vi "PJVS.vi"(3 "Trim current (A) (+- 0.002)":dbl, 4 "Samples (2) (2 - 256)":i32=2 min=2 max=256, 5 "Frequency  (0 Hz) (0, 0.5 - 10e3)":dbl, 6 "Waveform (Sinewave)":T2, 7 "Voltage (0 V DC/RMS) (DC: +- 10.1, AC: 0 - 7.2)":dbl, 8 "error in (no error)":errorcluster) -> (0 "error out":errorcluster, 2 "PJVS Voltages":T1={"DC Voltage (S)"=nan, "AC Josephson Voltage RMS (V)"=nan, "Number of steps"=-1, "AC Voltages (V)"=[]} {"AC Voltages (V)" format="%#_10g"; "AC Josephson Voltage RMS (V)" format="%#_10g"; "DC Voltage (S)" format="%#_10g"})   [LabVIEW 2019, in "ACSVcontrol-driver.lvlib"]
doc: "Sets PJVS voltage(s). If frequency is nonzero, the AC mode is supposed. Samples sets the number of steps into which the waveform is divided. Output is a structure with DC voltage or AC voltages and steps."
uses:
  ACSVcontrol-driver.lvlib
  Type Definitions/Waveform.ctl
  Type Definitions/PJVS Voltages.ctl
  Private/Type definitions/Command.ctl
  Private/Type definitions/Status.ctl
  Private/Type definitions/Instruction.ctl
  Private/Globals.vi
  <vilib>/Utility/error.llb/Error Cluster From Error Code.vi
  <vilib>/ErrorRing/Error Ring.xnode
panel:
  in  "number format string":string="%.6f"
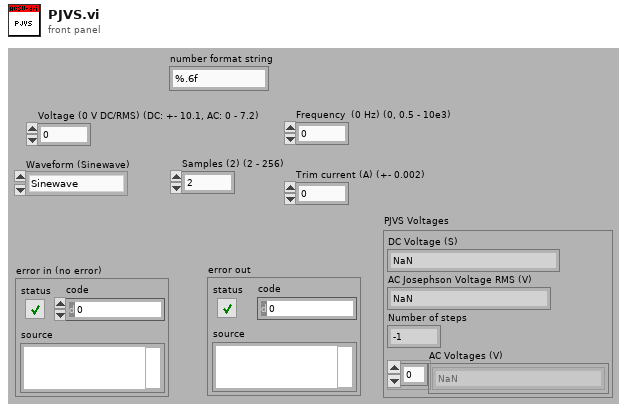
[diagram p1: front panel]
types:
  T1 = typedef "ACSVcontrol-driver.lvlib/PJVS Voltages.ctl" = cluster{"DC Voltage (S)":dbl, "AC Josephson Voltage RMS (V)":dbl, "Number of steps":i32, "AC Voltages (V)":dbl[]}
  T2 = typedef "ACSVcontrol-driver.lvlib/Waveform.ctl" = enum16{"Sinewave", "Triangle", "Sawtooth", "Rectangle", "Arbitrary"}
  T3 = typedef "ACSVcontrol-driver.lvlib/Status.ctl" = enum16{"waiting", "processing", "error command", "Set_PJVS-Done", "Set_Mux-Done", "Set_Mux-Error", "Set_57XX-Done", "Set_57XX-Error", "Set_Gen-Done", "Set_Gen-Error", "Set_Synthesizer-Done", "Set_Synthesizer-Error", "Read_Nano-Done", "Read_Sampler-Done", "Read_Sampler-Error", "Read_Sensors-Done"}
  T4 = typedef "ACSVcontrol-driver.lvlib/Command.ctl" = enum16{"Set_PJVS", "Set_Mux", "Set_57XX", "Set_Gen", "Set_Synthesizer", "Read_Nulldetector", "Read_Sampler", "Read_Sensors"}
  T5 = typedef "ACSVcontrol-driver.lvlib/Instruction.ctl" = enum16{"dummy - do not use", "Send Command", "Read Result", "Ask Status"}
  T6 = typedef "ACSVcontrol-driver.lvlib/Timeouts.ctl" = cluster{"TCP Read & Write (ms)":i32, "Sensors readout":i32, "PJVS setup":i32, "Nullmeter readout":i32, "Multiplexer setup":i32, "57XX setup":i32, "Generator setup":i32, "Synthesizer setup":i32, "Sampler readout":i32}
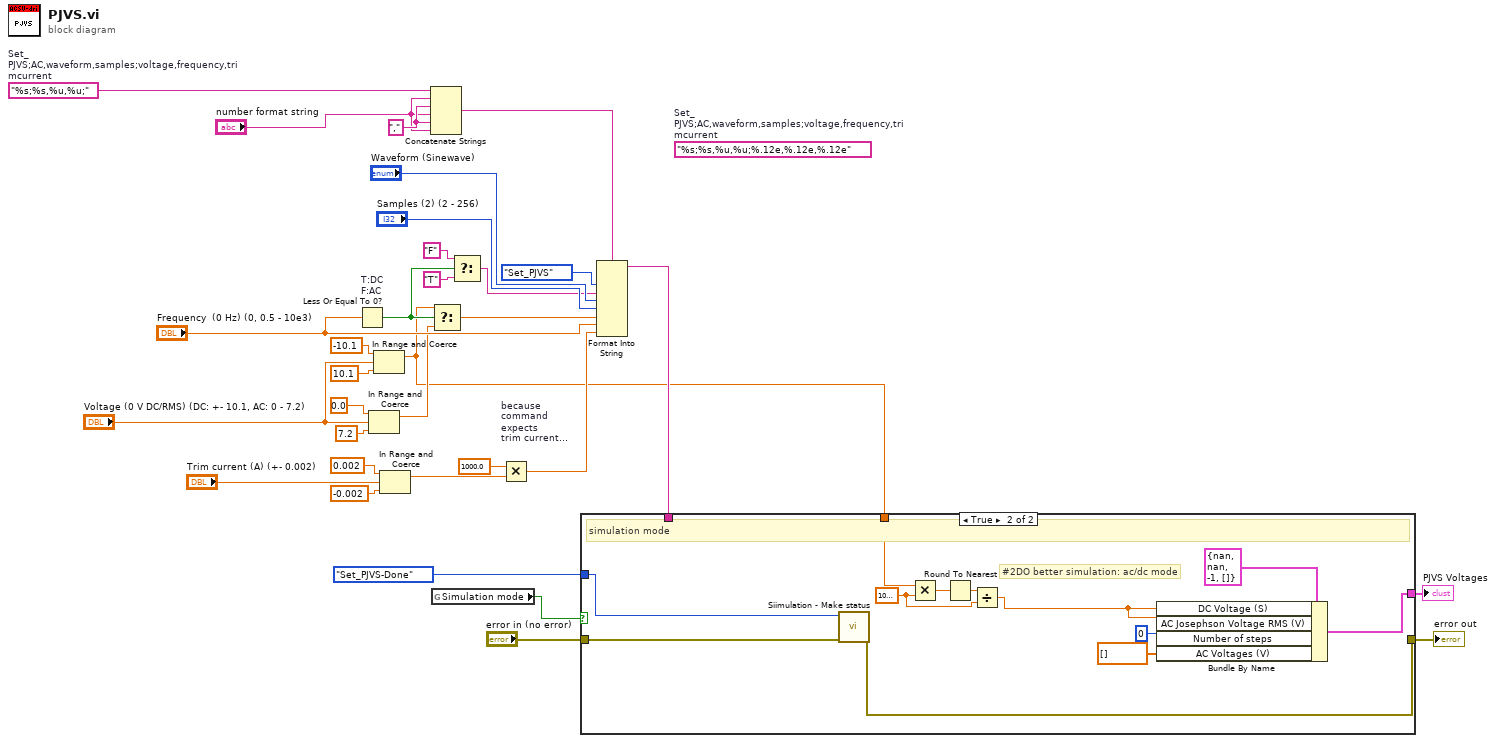
[diagram p0: block diagram]
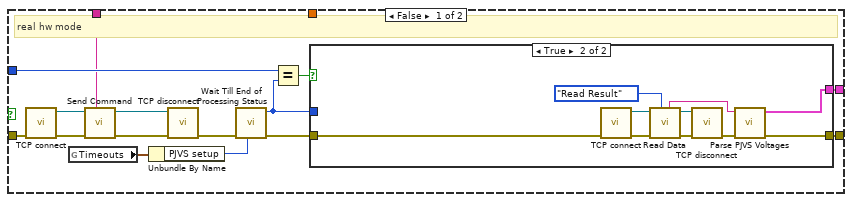
[diagram p2: hidden frame]
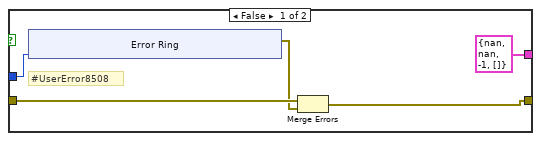
[diagram p3: hidden frame]
diagram:
  w9 = "%s;%s,%u,%u;"  # Set_PJVS;AC,waveform,samples;voltage,frequency,trimcurrent
  w11 = "," ("string")
  (unwired) "%s;%s,%u,%u;%.12e,%.12e,%.12e"  # Set_PJVS;AC,waveform,samples;voltage,frequency,trimcurrent
  n1 = Less Or Equal To 0? "T:DC\nF:AC"(x="Frequency  (0 Hz) (0, 0.5 - 10e3)") -> (x <= 0?=w16:bool)
  n2 = In Range and Coerce(upper limit=0.0, x="Voltage (0 V DC/RMS) (DC: +- 10.1, AC: 0 - 7.2)", lower limit=7.2) -> (coerced(x)=w2:dbl)  [unwired: 1 out]
  n3 = In Range and Coerce(upper limit=-10.1, x="Voltage (0 V DC/RMS) (DC: +- 10.1, AC: 0 - 7.2)", lower limit=10.1) -> (coerced(x)=w1:dbl)  [unwired: 1 out]
  n4 = In Range and Coerce(upper limit=0.002, x="Trim current (A) (+- 0.002)", lower limit=-0.002) -> (coerced(x)=w5:dbl)  [unwired: 1 out]
  n5 = Concatenate Strings(w9, "number format string", w11, "number format string", w11, "number format string") -> (w8:string)
  n6 = Select(t=w1, s=w16, f=w2) -> (s? t:f=w15:dbl)
  n7 = global read "Globals.vi" "Simulation mode"() -> (w3:bool)
  n8 = Select(t="F" ("format string"), s=w16, f="T" ("format string")) -> (s? t:f=w26:string)
  n9 = Multiply "because\ncommand\nexpects\ntrim current\nin miliampers"(x=1000.0, y=w5) -> (x*y=w4:dbl)
  n10 = Format Into String(format string=w8, Command."Set_PJVS" ("Command"), w26, "Waveform (Sinewave)", "Samples (2) (2 - 256)", w15, "Frequency  (0 Hz) (0, 0.5 - 10e3)", w4) -> (resulting string=w7:string)  [unwired: 2 in, 1 out]
  n11 = case shown="True" w3 {
    tunnel: "error in (no error)" -> [w43 w81]
    tunnel: Status."Set_PJVS-Done" ("x") -> [w40 w79]
    tunnel: [w37 w80] -> w13
    tunnel: [w36 w77] -> w12
    tunnel: w7 -> [w33 _]
    tunnel: w1 -> [_ w74]
    frame False {
      # "real hw mode"
      n12 = call "TCP connect.vi"("error in (no error)"=w43) -> ("error out"=w46:errorcluster, "connection ID"=w47:refnum<k5>)  [unwired: 9 in]
      n13 = global read "Globals.vi" "Timeouts"() -> (w34:T6)
      n14 = call "Send Command.vi"("Command"=w33, "error in (no error)"=w46, "connection ID"=w47) -> ("error out"=w45:errorcluster, "connection ID out"=w44:refnum<k5>)  [unwired: 7 in]
      n15 = Unbundle By Name(w34) -> ("PJVS setup"=w35:i32)
      n16 = call "TCP disconnect.vi"("error in (no error)"=w45, "connection ID"=w44) -> ("error out"=w38:errorcluster)  [unwired: 9 in]
      n17 = call "Wait Till End of Processing Status.vi"("Loop Timeout (ms) (5000)"=w35, "error in (no error)"=w38) -> ("error out"=w39:errorcluster, "Last Status"=w42:T3)  [unwired: 8 in]
      n18 = Equal?(x=w40, y=w42) -> (x = y?=w41:bool)
      n19 = case shown="True" w41 {
        tunnel: w39 -> [w52 w67]
        tunnel: [w49 w63] -> w37
        tunnel: w42 -> [w51 _]
        tunnel: [T1 {"DC Voltage (S)"=nan, "AC Josephson Voltage RMS (V)"=nan, "Number of steps"=-1, "AC Voltages (V)"=[]} ("PJVS Voltages") w62] -> w36
        frame False {
          # "#UserError8508"
          n20 = xnode "Error Ring"("parameter 0"=w51) -> ("error out"=w50:errorcluster)
          n21 = Merge Errors(w52, w50) -> (w49:errorcluster)
        }
        frame True {
          n22 = call "TCP connect.vi"("error in (no error)"=w67) -> ("error out"=w66:errorcluster, "connection ID"=w65:refnum<k5>)  [unwired: 9 in]
          n23 = call "Read Data.vi"("Instruction"=Instruction."Read Result", "error in (no error)"=w66, "connection ID"=w65) -> ("error out"=w69:errorcluster, "connection ID out"=w68:refnum<k5>, "Data"=w61:string)  [unwired: 6 in]
          n24 = call "TCP disconnect.vi"("error in (no error)"=w69, "connection ID"=w68) -> ("error out"=w64:errorcluster)  [unwired: 9 in]
          n25 = call "Parse PJVS Voltages.vi"("error in"=w64, "Data"=w61) -> ("error out"=w63:errorcluster, "PJVS Voltages"=w62:T1)  [unwired: 8 in]
        }
      }
    }
    frame True {
      w71 = 10000.0 ("y")
      # "#2DO better simulation: ac/dc mode"
      # "simulation mode"
      n26 = call "Siimulation - Make status.vi"("error in (no error)"=w81, "Status"=w79) -> ("error out"=w80:errorcluster)  [unwired: 8 in, 1 out]
      n27 = Multiply(x=w74, y=w71) -> (x*y=w73:dbl)
      n28 = Round To Nearest(number=w73) -> (nearest integer value=w72:dbl)
      n29 = Divide(x=w72, y=w71) -> (x/y=w70:dbl)
      n30 = Bundle By Name(cluster=T1 {"DC Voltage (S)"=nan, "AC Josephson Voltage RMS (V)"=nan, "Number of steps"=-1, "AC Voltages (V)"=[]} ("PJVS Voltages"), "DC Voltage (S)"=w70, "AC Josephson Voltage RMS (V)"=w70, "Number of steps"=0, "AC Voltages (V)"=dbl[] []) -> (w77:T1)
    }
  }
  "error out" <- w13
  "PJVS Voltages" <- w12
